vi "fromXML.vi"(8 "error in (no error)":errorcluster, 9 "xmlPath":string, 10 "channel_configXML":refnum<class "NativeXML.lvclass">, 11 "Channel in":refnum<class "Channel.lvclass">) -> (0 "error out":errorcluster, 3 "Channel out":refnum<class "Channel.lvclass">)   [LabVIEW 2011, in "Tools.lvlib" / "DatabaseHelpers.lvlib" / "Channel.lvclass"]
uses:
  Channel.lvclass
  NativeXML/NativeXML.lvclass
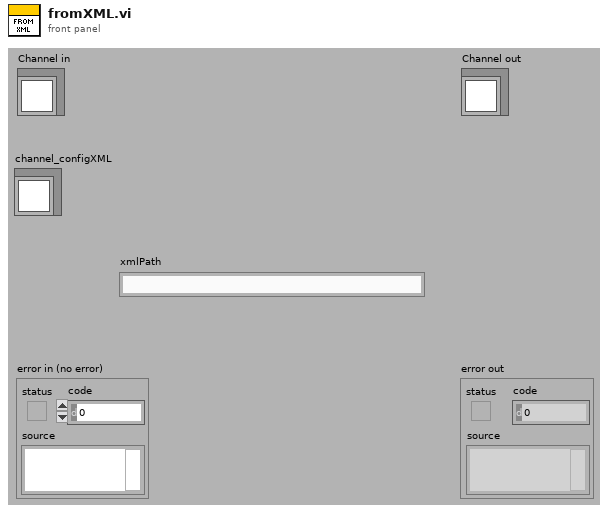
[diagram p1: front panel]
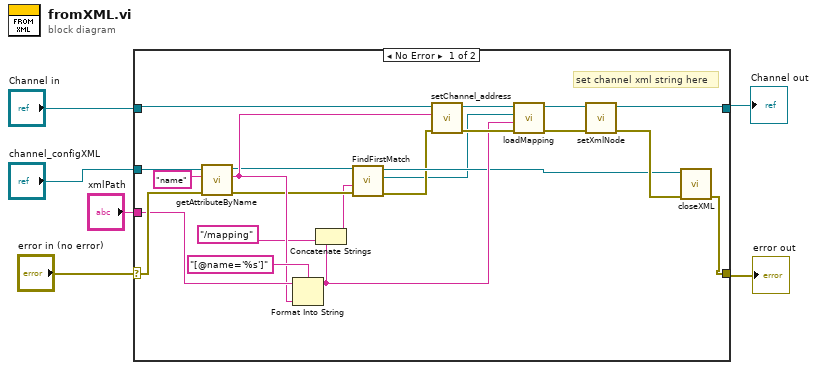
[diagram p0: block diagram]
diagram:
  n1 = case shown="No Error" "error in (no error)" {
    selector: "error in (no error)" -> [w21 w30]
    tunnel: [w18 w30] -> w5
    tunnel: [w24 w29] -> w3
    tunnel: "Channel in" -> [w28 w29]
    tunnel: "channel_configXML" -> [w22 _]
    tunnel: "xmlPath" -> [w17 _]
    frame No Error {
      # "set channel xml string here"
      n2 = call "getAttributeByName.vi"("error in (no error)"=w21, "name"="name", "NativeXML in"=w22) -> ("error out"=w12:errorcluster, "Attribute String"=w15:string, "NativeXML out"=w11:refnum<class "NativeXML.lvclass">)  [unwired: 6 in]
      n3 = Format Into String(format string="[@name='%s']", initial string=w17, w15) -> (resulting string=w14:string)  [unwired: 1 in, 1 out]
      n4 = Concatenate Strings(w14, "/mapping") -> (w7:string)
      n5 = call "FindFirstMatch.vi"("error in (no error)"=w12, "xPath"=w7, "NativeXML in"=w11) -> ("error out"=w9:errorcluster, "NativeXML match"=w8:refnum<class "NativeXML.lvclass">, "NativeXML out"=w10:refnum<class "NativeXML.lvclass">)  [unwired: 6 in]
      n6 = call "setChannel_address.vi"("error in (no error)"=w9, "channel_address"=w15, "Channel.lvclass in"=w28) -> ("error out"=w25:errorcluster, "Channel.lvclass out"=w27:refnum<class "Channel.lvclass">)  [unwired: 7 in]
      n7 = call-dynamic "loadMapping.vi"("error in (no error)"=w25, "xmlPath"=w14, "channel_configXML"=w8, "Channel in"=w27) -> ("error out"=w20:errorcluster, "Channel out"=w26:refnum<class "Channel.lvclass">)  [unwired: 6 in]
      n8 = call "setXmlNode.vi"("error in (no error)"=w20, "Channel.lvclass in"=w26) -> ("error out"=w19:errorcluster, "Channel.lvclass out"=w24:refnum<class "Channel.lvclass">)  [unwired: 8 in]
      n9 = call "closeXML.vi"("error in (no error)"=w19, "NativeXML in"=w10) -> ("error out"=w18:errorcluster)  [unwired: 9 in]
    }
    frame Error {
    }
  }
  "error out" <- w5
  "Channel out" <- w3
